vi "XY Graph Shift Plot (Core).vi"(6 "Plot Shift Parameters":T2 caption="Decay Shift Parameters", 7 "Time-Gated Reference Decay":cluster{"t Array":dbl[], "I Array":dbl[]}, 8 "error in (no error)":errorcluster, 11 "Decay in":T1) -> (0 "error out":errorcluster, 1 "Shift (ns)":dbl, 3 "Decay out":T1)   [LabVIEW 2021, in "XY Graph Add-Ons.lvlib"]
uses:
  XY Graph Add-Ons.lvlib
  XY Graph Plot Shift Parameters.ctl
  XY Graph Plot Shift Method.ctl
  aa23abca-14a8-4031-8085-0911445f1ce7.vi
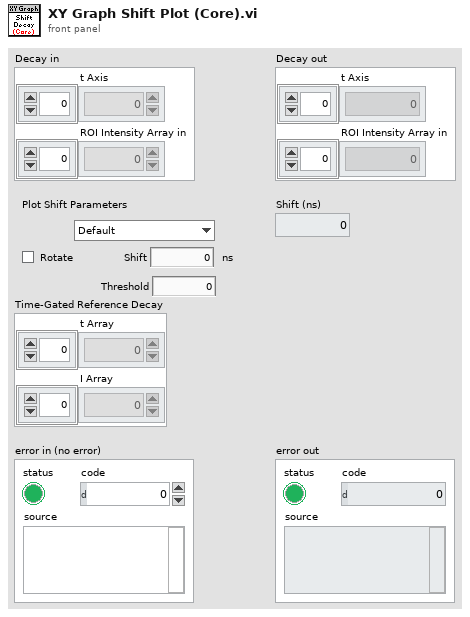
[diagram p1: front panel]
types:
  T1 = cluster{"t Axis":dbl[], "ROI Intensity Array in":dbl[]}
  T2 = typedef "XY Graph Add-Ons.lvlib/XY Graph Plot Shift Parameters.ctl" = cluster{"Type":T3, "Shift":dbl[unit], "Threshold":dbl, "Rotate":bool}
  T3 = typedef "XY Graph Add-Ons.lvlib/XY Graph Plot Shift Method.ctl" = enum16{"Default", "CFD", "Threshold", "Cross-Correlation"}
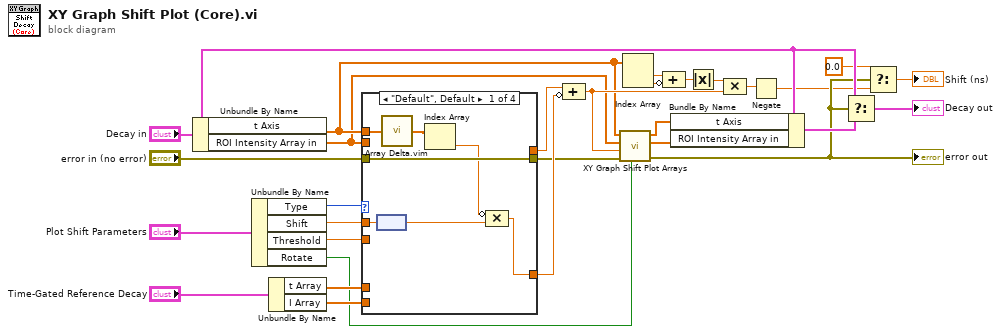
[diagram p0: block diagram]
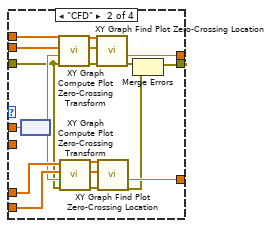
[diagram p2: hidden frame]
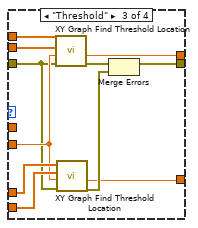
[diagram p3: hidden frame]
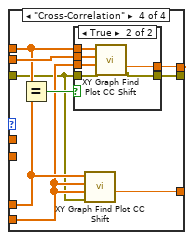
[diagram p4: hidden frame]
diagram:
  n1 = Unbundle By Name("Decay in") -> ("t Axis"=w23:dbl[], "ROI Intensity Array in"=w22:dbl[])
  n2 = Unbundle By Name("Plot Shift Parameters") -> ("Type"=w10:T3, "Shift"=w11:dbl[unit], "Threshold"=w12:dbl, "Rotate"=w1:bool)
  n3 = Unbundle By Name("Time-Gated Reference Decay") -> ("t Array"=w14:dbl[], "I Array"=w15:dbl[])
  n4 = case shown="\"Default\", Default" w10 {
    tunnel: [_ w47 w62 w71] -> w17
    tunnel: w11 -> [w35 w52 _ _]
    tunnel: w23 -> [w34 w54 w65 w73]
    tunnel: w22 -> [_ w53 w64 w74]
    tunnel: w12 -> [_ _ w59 _]
    tunnel: w14 -> [_ w44 w61 w69]
    tunnel: w15 -> [_ w43 w60 w68]
    tunnel: "error in (no error)" -> [w36 w41 w58 w67]
    tunnel: [w36 w38 w57 w70] -> w16
    tunnel: [w31 w39 w55 w66] -> w18
    frame "Default", Default {
      n5 = node(w35) -> (w33:dbl)
      n6 = call "Array Delta.vim"("A[i]"=w34) -> ("A[i+1]-A[i]"=w32:dbl[])  [unwired: 8 in]
      n7 = Index Array(array=w32) -> (element=w30:dbl)  [unwired: 1 in]
      n8 = Compound Arithmetic op=MULTIPLY(invert w30, w33) -> (w31:dbl)
    }
    frame "CFD" {
      n9 = node(w52) -> (w42:dbl)
      n10 = call "XY Graph Compute Plot Zero-Crossing Transform.vi"("Error In"=w41, "Shift"=w42, "IRF Array in"=w53, "t Array in"=w54) -> ("Error Out"=w49:errorcluster, "ZC IRF Array out"=w50:dbl[], "t Array (dup) out"=w51:dbl[])  [unwired: 5 in]
      n11 = call "XY Graph Compute Plot Zero-Crossing Transform.vi"("Error In"=w41, "Shift"=w42, "IRF Array in"=w43, "t Array in"=w44) -> ("Error Out"=w40:errorcluster, "ZC IRF Array out"=w46:dbl[], "t Array (dup) out"=w45:dbl[])  [unwired: 5 in]
      n12 = call "XY Graph Find Plot Zero-Crossing Location.vi"("Error In"=w49, "Y Array"=w50, "X Array"=w51) -> ("Error Out"=w48:errorcluster, "Location Index"=w47:dbl)  [unwired: 6 in, 1 out]
      n13 = call "XY Graph Find Plot Zero-Crossing Location.vi"("Error In"=w40, "Y Array"=w46, "X Array"=w45) -> ("Error Out"=w37:errorcluster, "Location Index"=w39:dbl)  [unwired: 6 in, 1 out]
      n14 = Merge Errors(w48, w37) -> (w38:errorcluster)
    }
    frame "Threshold" {
      n15 = call "XY Graph Find Threshold Location.vi"("Error In"=w58, "Threshold"=w59, "Y Array"=w64, "X Array"=w65) -> ("Error Out"=w63:errorcluster, "Location Index"=w62:dbl)  [unwired: 5 in, 1 out]
      n16 = call "XY Graph Find Threshold Location.vi"("Error In"=w58, "Threshold"=w59, "Y Array"=w60, "X Array"=w61) -> ("Error Out"=w56:errorcluster, "Location Index"=w55:dbl)  [unwired: 5 in, 1 out]
      n17 = Merge Errors(w63, w56) -> (w57:errorcluster)
    }
    frame "Cross-Correlation" {
      n18 = Equal?(x=w73, y=w69) -> (x = y?=w72:bool)
      n19 = case shown="True" w72 {
        tunnel: w74 -> [_ w81]
        tunnel: w73 -> [_ w80]
        tunnel: w68 -> [_ w79]
        tunnel: [_ w76] -> w71
        tunnel: w67 -> [w75 w78]
        tunnel: [w75 w77] -> w70
        frame False {
        }
        frame True {
          n20 = call "XY Graph Find Plot CC Shift.vi"("Error In"=w78, "Ref Array"=w79, "Y Array"=w81, "X Array"=w80) -> ("Error Out"=w77:errorcluster, "Shift (Index Unit)"=w76:dbl)  [unwired: 5 in, 1 out]
        }
      }
      n21 = call "XY Graph Find Plot CC Shift.vi"("Error In"=w67, "Ref Array"=w68, "Y Array"=w68, "X Array"=w69) -> ("Shift (Index Unit)"=w66:dbl)  [unwired: 5 in, 2 out]
    }
  }
  n22 = Compound Arithmetic op=ADD(w17, invert w18) -> (w27:dbl)
  n23 = call "XY Graph Shift Plot Arrays.vi"("Rotate"=w1, "Error In"=w16, "Shift [index value] (0)"=w27, "Y Array"=w22, "X Array"=w23) -> ("Error Out"=w5:errorcluster, "Y Array (shifted)"=w24:dbl[], "X Array (out)"=w25:dbl[])  [unwired: 4 in]
  "error out" <- w5
  n24 = Index Array(array=w23) -> (element #1=w19:dbl, element #2=w20:dbl)  [unwired: 2 in]
  n25 = Compound Arithmetic op=ADD(w19, invert w20) -> (w21:dbl)
  n26 = Bundle By Name(cluster="Decay in", "t Axis"=w25, "ROI Intensity Array in"=w24) -> (w8:T1)
  n27 = Absolute Value(x=w21) -> (abs(x)=w9:dbl)
  n28 = Compound Arithmetic op=MULTIPLY(w9, w27) -> (w26:dbl)
  n29 = Negate(x=w26) -> (-x=w4:dbl)
  n30 = Select(t="Decay in", s=w5, f=w8) -> (s? t:f=→"Decay out":T1)
  n31 = Select(t=0.0, s=w5, f=w4) -> (s? t:f=→"Shift (ns)":dbl)
